vi "Configure Position Offset.vi"(8 "error in (no error)":errorcluster, 10 "CCW Position Offset (0.0 rad)":dbl, 11 "Hitec HS400 Series in":refnum<class "Hitec HS400 Series.lvclass">) -> (0 "error out":errorcluster, 3 "Hitec HS400 Series out":refnum<class "Hitec HS400 Series.lvclass">)   [LabVIEW 2013, in "Hitec HS400 Series.lvclass"]
doc: "Configures the counterclockwise software position offset."
uses:
  Hitec HS400 Series.lvclass
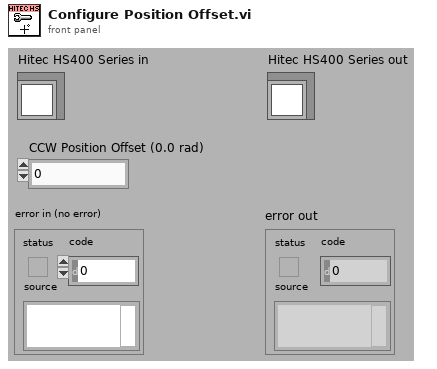
[diagram p1: front panel]
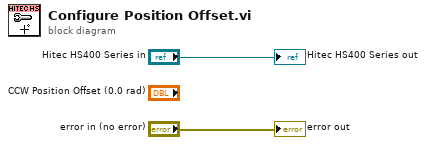
[diagram p0: block diagram]
diagram:
  "error out" <- "error in (no error)"
  "Hitec HS400 Series out" <- "Hitec HS400 Series in"
